vi "Check Available Submission.vi"(8 "error in (no error)":errorcluster, 10 "Scorer In":refnum<class "Scorer.lvclass">, 11 "SOL-Server in":refnum<class "SOL-Server.lvclass">) -> (0 "error out":errorcluster, 2 "Scorer":refnum<class "Scorer.lvclass">, 3 "SOL-Server out":refnum<class "SOL-Server.lvclass">)   [LabVIEW 2020, in "Summer of LabVIEW.lvlib" / "SOL-Server.lvclass"]
uses:
  SOL-Server.lvclass
  Scorer/Scorer.lvclass
  SOL-Server.lvclass/SOL-Server.ctl
  Submission DB/Submission DB.lvclass
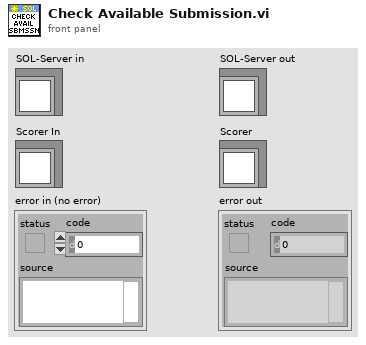
[diagram p1: front panel]
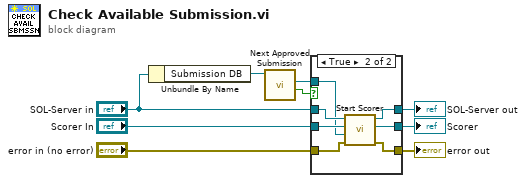
[diagram p0: block diagram]
diagram:
  n1 = Unbundle By Name("SOL-Server in") -> ("Submission DB"=w9:refnum<class "Submission DB.lvclass">)
  n2 = call "Next Approved Submission.vi"("Submission DB in"=w9) -> ("Found?"=w8:bool, "Submission"=w7:refnum<class "Submission.lvclass">)  [unwired: 7 in, 2 out]
  n3 = case shown="True" w8 {
    tunnel: w7 -> [_ w13]
    tunnel: "Scorer In" -> [w12 w19]
    tunnel: [w12 w16] -> w5
    tunnel: "error in (no error)" -> [w11 w15]
    tunnel: [w11 w14] -> w3
    tunnel: "SOL-Server in" -> [w10 w18]
    tunnel: [w10 w17] -> w1
    frame False {
    }
    frame True {
      n4 = call "Start Scorer.vi"("error in (no error)"=w15, "Submission"=w13, "Scorer In"=w19, "SOL-Server in"=w18) -> ("error out"=w14:errorcluster, "Scorer"=w16:refnum<class "Scorer.lvclass">, "SOL-Server out"=w17:refnum<class "SOL-Server.lvclass">)  [unwired: 5 in]
    }
  }
  "error out" <- w3
  "SOL-Server out" <- w1
  "Scorer" <- w5
